vi "LEBITVacuum.SetPLCLL.vi"(0 "i ref in":refnum<vi>, 2 "i attribute in":T1={"setValuePLC"=[], "nickNames"=[], "setValuePLCServiceID"=[], "monValuePLC"=[], "SetValueServiceID"=[], "MonValueServiceID"=[], "SetValue"=[], "AllPLCValues"=[], "CondSpecial2DArray"=[], "CondSpecialIndex"=[], "ReasonForLocking"="", "ReasonForLockingID"=0, "enableValuePLC"=[], "OverwriteCloseSafetyPLC"=[], "OverwriteOpenSafetyPLC"=[], "OverwriteCloseSafetyPLCServiceID"=[], "OverwriteOpenSafetyPLCServiceID"=[], "MKS Address Array"=[], "MKS MeasurementServiceID"=[], "MKS Measurement"=[], "CRYO Measurement"=[], "CRYO MeasurementServiceID"=[], "Special"=[], "Start Date"="", "MKS VISA resource"="COM13", "CRYO VISA resource"="COM13"}, 3 "SetValue":i16, 4 "index of element":i32, 5 "error IO":errorcluster) -> (14 "i ref out":refnum<vi>, 15 "i attribute out":T1={"setValuePLC"=[], "nickNames"=[], "setValuePLCServiceID"=[], "monValuePLC"=[], "SetValueServiceID"=[], "MonValueServiceID"=[], "SetValue"=[], "AllPLCValues"=[], "CondSpecial2DArray"=[], "CondSpecialIndex"=[], "ReasonForLocking"="", "ReasonForLockingID"=0, "enableValuePLC"=[], "OverwriteCloseSafetyPLC"=[], "OverwriteOpenSafetyPLC"=[], "OverwriteCloseSafetyPLCServiceID"=[], "OverwriteOpenSafetyPLCServiceID"=[], "MKS Address Array"=[], "MKS MeasurementServiceID"=[], "MKS Measurement"=[], "CRYO Measurement"=[], "CRYO MeasurementServiceID"=[], "Special"=[], "Start Date"="", "MKS VISA resource"="COM13", "CRYO VISA resource"="COM13"}, 19 "error out":errorcluster)   [LabVIEW 2014, in "LEBITVacuum.lvlib"]
uses:
  LEBITVacuum.lvlib
  LEBITVacuum.i attribute.ctl
  CSlibraries/UtilityLib/UtilityLib.valueStatus.ctl
  CSlibraries-extern/DimLVEvent/LVDimInterface/LVDimInterface.lvlib
  CSCore/CSSystem/CoreLib/CoreLib.lvlib
  CSlibraries/UtilityLib/UtilityLib.lvlib
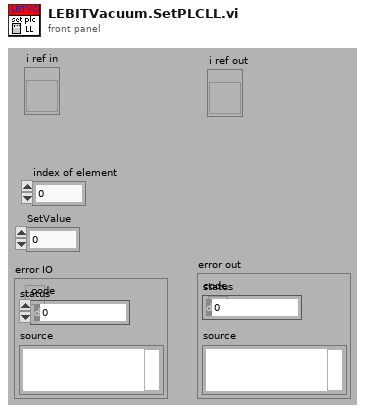
[diagram p1: front panel]
types:
  T1 = typedef "LEBITVacuum.lvlib/LEBITVacuum.i attribute.ctl" = cluster{"setValuePLC":string[], "nickNames":string[], "setValuePLCServiceID":i32[], "monValuePLC":string[], "SetValueServiceID":i32[], "MonValueServiceID":i32[], "SetValue":i16[], "AllPLCValues":string[], "CondSpecial2DArray":string[][], "CondSpecialIndex":i32[], "ReasonForLocking":string, "ReasonForLockingID":i32, "enableValuePLC":string[], "OverwriteCloseSafetyPLC":string[], "OverwriteOpenSafetyPLC":string[], "OverwriteCloseSafetyPLCServiceID":i32[], "OverwriteOpenSafetyPLCServiceID":i32[], "MKS Address Array":i32[][], "MKS MeasurementServiceID":i32[], "MKS Measurement":string[], "CRYO Measurement":string[][], "CRYO MeasurementServiceID":i32[], "Special":string[], "Start Date":string, "MKS VISA resource":refnum<visa-resource-name>, "CRYO VISA resource":refnum<visa-resource-name>}
  T2 = typedef "UtilityLib.lvlib/UtilityLib.valueStatus.ctl" = enum16{"no info available", "stand by/off", "on", "warning", "alarm/malfunction", "not implemented", "user action required", "important information", "system default", "control default", "indicator default", "button default"}
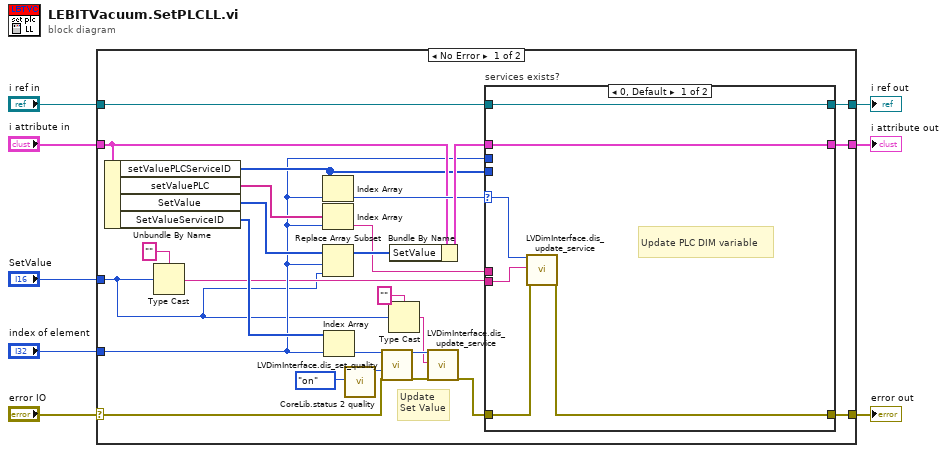
[diagram p0: block diagram]
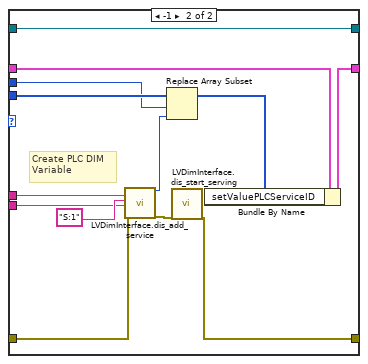
[diagram p2: hidden frame]
diagram:
  n1 = case shown="No Error" "error IO" {
    selector: "error IO" -> [w18 w54]
    tunnel: "index of element" -> [w12 _]
    tunnel: "i attribute in" -> [w17 w55]
    tunnel: [w27 w55] -> w6
    tunnel: [w26 w54] -> w5
    tunnel: [w25 w56] -> w4
    tunnel: "i ref in" -> [w23 w56]
    tunnel: "SetValue" -> [w9 _]
    frame No Error {
      # "Update\nSet Value"
      n2 = Unbundle By Name(w17) -> ("setValuePLCServiceID"=w16:i32[], "setValuePLC"=w15:string[], "SetValue"=w13:i16[], "SetValueServiceID"=w14:i32[])
      n3 = Type Cast(type="", x=w9) -> (*(type *) &x=w10:string)
      n4 = Index Array(array=w16, index=w12) -> (element=w21:i32)
      n5 = Index Array(array=w15, index=w12) -> (element=w22:string)
      n6 = Replace Array Subset(array=w13, new element=w9, index=w12) -> (w34:i16[])
      n7 = Index Array(array=w14, index=w12) -> (element=w30:i32)
      n8 = call "CoreLib.status 2 quality.vi"("valueStatus"=UtilityLib.valueStatus."on") -> ("quality"=w31:i32)  [unwired: 18 in]
      n9 = call "LVDimInterface.dis_set_quality.vi"("my_serviceID"=w30, "quality"=w31, "error in (no error)"=w18) -> ("my_serviceID (out)"=w29:i32, "error out"=w28:errorcluster)  [unwired: 15 in]
      n10 = Type Cast(type="", x=w9) -> (*(type *) &x=w20:string)
      n11 = Bundle By Name(cluster=w17, "SetValue"=w34) -> (w33:T1)
      n12 = call "LVDimInterface.dis_update_service.vi"("my_serviceID"=w29, "data"=w20, "error in (no error)"=w28) -> ("error out"=w24:errorcluster)  [unwired: 14 in, 2 out]
      n13 = case "services exists?" shown="0, Default" w21 {
        selector: w21 -> [w40 _]
        tunnel: w10 -> [w39 w41]
        tunnel: w22 -> [_ w42]
        tunnel: w23 -> [w38 w48]
        tunnel: [w38 w48] -> w25
        tunnel: w24 -> [w36 w46]
        tunnel: w16 -> [_ w53]
        tunnel: [w35 w44] -> w26
        tunnel: w12 -> [_ w52]
        tunnel: w33 -> [w37 w49]
        tunnel: [w37 w47] -> w27
        frame 0, Default {
          # "Update PLC DIM variable"
          n14 = call "LVDimInterface.dis_update_service.vi"("my_serviceID"=w40, "data"=w39, "error in (no error)"=w36) -> ("error out"=w35:errorcluster)  [unwired: 14 in, 2 out]
        }
        frame -1 {
          # "Create PLC DIM\nVariable"
          n15 = call "LVDimInterface.dis_add_service.vi"("serviceName"=w42, "typeDescriptor"="S:1", "data"=w41, "error in (no error)"=w46) -> ("my_serviceID"=w51:i32, "error out"=w45:errorcluster)  [unwired: 14 in]
          n16 = Replace Array Subset(array=w53, new element=w51, index=w52) -> (w50:i32[])
          n17 = call "LVDimInterface.dis_start_serving.vi"("error in (no error)"=w45) -> ("error out"=w44:errorcluster)  [unwired: 17 in, 1 out]
          n18 = Bundle By Name(cluster=w49, "setValuePLCServiceID"=w50) -> (w47:T1)
        }
      }
    }
    frame Error {
    }
  }
  "i attribute out" <- w6
  "error out" <- w5
  "i ref out" <- w4
